vi "Make the Rock to Fall.vi"(0 "Chamber in":u32[][](array[colorbox]), 3 "Rock Position in Chamber in":i32=3, 4 "Rock in":u32[][](array[colorbox])) -> (1 "Settled ?":bool=TRUE, 2 "Chamber out":u32[][](array[colorbox]), 5 "Rock Position in Chamber out":i32=3)   [LabVIEW 2020, in "AoC 2022.lvlib"]
uses:
  AoC 2022.lvlib
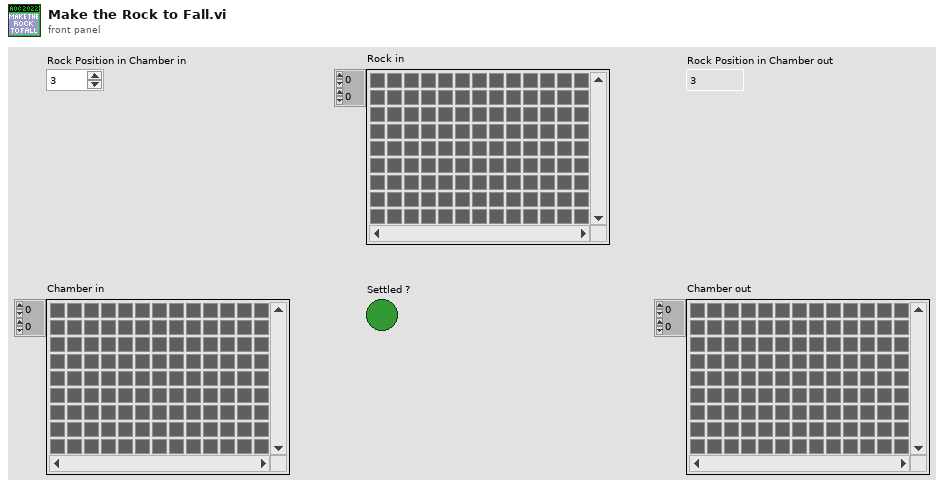
[diagram p1: front panel]
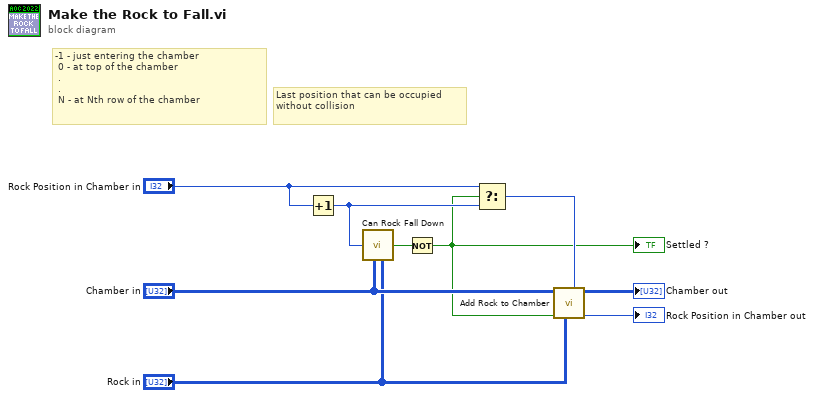
[diagram p0: block diagram]
diagram:
  # "Last position that can be occupied without collision"
  # "-1 - just entering the chamber\n 0 - at top of the chamber\n .\n .\n N - at Nth row of the chamber"
  n1 = Increment(x="Rock Position in Chamber in") -> (x+1=w6:i32)
  n2 = call "Can Rock Fall Down.vi"("Position in Chamber to Check"=w6, "Chamber"="Chamber in", "Rock"="Rock in") -> ("Can Rock Fall Down ?"=w5:bool)
  n3 = Not(x=w5) -> (.not. x?=w3:bool)
  "Settled ?" <- w3
  n4 = Select(t="Rock Position in Chamber in", s=w3, f=w6) -> (s? t:f=w4:i32)
  n5 = call "Add Rock to Chamber.vi"("Rock Position in Chamber in"=w4, "Rock"="Rock in", "include Clipped Parts ? (F)"=w3, "Chamber in"="Chamber in") -> ("Rock Position in Chamber out"=→"Rock Position in Chamber out":i32, "Chamber out"=→"Chamber out":u32[][])  [unwired: 4 in]
